vi "Begin.vi"(8 "error in":errorcluster) -> (0 "error out":errorcluster)   [LabVIEW 2014]
doc: "Called before other user functions, this VI is expected to open initial I/O refnums, load in file data, and do all program initialization. Notice that the <B>error out</B> terminal is simply used for data flow. Wiring it to other structures or subVIs ensures that this VI runs first."
uses:
  <vilib>/Rock Robotics/SystemInterfaces/DIO/FPGA_DIOPWMChannel.ctl
  <vilib>/Rock Robotics/WPI/SafetyOutput/WPI_SafetyOutputConfigMenu.ctl
  <vilib>/Rock Robotics/WPI/DriverStation/WPI_DriverStationRobotMode2.ctl
  <vilib>/Rock Robotics/WPI/Joystick/WPI_JoystickDeviceEnum.ctl
  <vilib>/Rock Robotics/SystemInterfaces/i2clib/i2c_bus.ctl
  <vilib>/Rock Robotics/SystemInterfaces/Typedef/FPGA_TypedefDigitalModule.ctl
  <vilib>/Rock Robotics/WPI/RobotDrive/WPI_RobotDriveOpen2MotorWithTalon.vi
  Robot Global Data.vi
  <vilib>/Rock Robotics/Network Tables/SD Write String Array.vi
panel:
  out "I2c Error":errorcluster
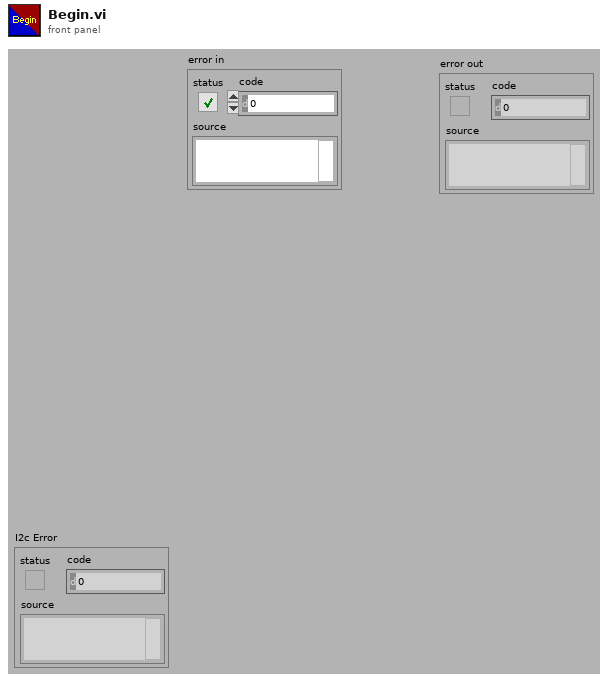
[diagram p1: front panel]
types:
  T1 = typedef "FPGA_TypedefDigitalModule.ctl" = enum16{"Controller 1"}
  T2 = typedef "i2c_bus.ctl" = enum16{"I2C On-Board", "I2C MXP", "Invalid"}
  T3 = typedef "WPI_JoystickDeviceEnum.ctl" = enum16{"USB 0", "USB 1", "USB 2", "USB 3", "USB 4", "USB 5"}
  T4 = typedef "WPI_DriverStationRobotMode2.ctl" = enum16{"Autonomous Disabled", "Autonomous Enabled", "Teleop Disabled", "Teleop Enabled", "Disconnected", "Finish", "Test Disabled", "Test Enabled", "Emergency Stopped"}
  T5 = typedef "WPI_SafetyOutputConfigMenu.ctl" = enum16{"Enable", "Disable"}
  T6 = typedef "FPGA_DIOPWMChannel.ctl" = enum8{"PWM 0", "PWM 1", "PWM 2", "PWM 3", "PWM 4", "PWM 5", "PWM 6", "PWM 7", "PWM 8", "PWM 9", "PWM MXP 0", "PWM MXP 1", "PWM MXP 2", "PWM MXP 3", "PWM MXP 4", "PWM MXP 5", "PWM MXP 6", "PWM MXP 7", "PWM MXP 8", "PWM MXP 9", "Invalid"}
  T7 = typedef "WPI_JoystickDevRef.ctl" = cluster{"Device":T3}
  T8 = typedef "WPI_RobotDriveDevRef.ctl" = cluster{"DevStatus":errorcluster, "Motors[]":T9[], "Square Inputs":bool, "Max Output":dbl}
  T9 = typedef "WPI_MotorControlDeviceRef.ctl" = cluster{"DeviceStatus":errorcluster, "Type":T10, "PWM":cluster{"Controller":T1, "PWM Channel":T6, "DeadBand":T11}, "CAN":cluster{"Device Number":u8, "Control Mode":T12, "Semaphore":T13, "Max Vout":dbl, "TalonSRX Control Mode":T14}, "Invert":bool, "TransformRef":T15, "InvTransformRef":T15}
  T10 = typedef "WPI_MotorControlType.ctl" = enum16{"PWM", "CAN", "CANTalonSRX"}
  T11 = typedef "WPI_PWMDeadband.ctl" = cluster{"Name":string, "maxPositivePwm":i32, "minPositivePwm":i32, "centerPwm":i32, "maxNegativePwm":i32, "minNegativePwm":i32, "angularRange":u16}
  T12 = typedef "WPI_CANJaguar_ControlMode.ctl" = enum8{"Percent VBus", "Current", "Speed", "Position", "Voltage"}
  T13 = typedef "Semaphore RefNum" = refnum<k1>
  T14 = typedef "WPI_CANTalonSRX_APIControlMode.ctl" = enum8{"Percent VBus", "Speed", "Position", "Slave", "Unchanged / Invalid"}
  T15 = typedef "WPI_PWMTransform_ConPane.ctl" = refnum<vi>
  T16 = typedef "WPI_I2CDevRef.ctl" = cluster{"DevStatus":errorcluster, "Controller":T1, "Device Address":u8, "Handle":i32, "I2C Bus":T2}
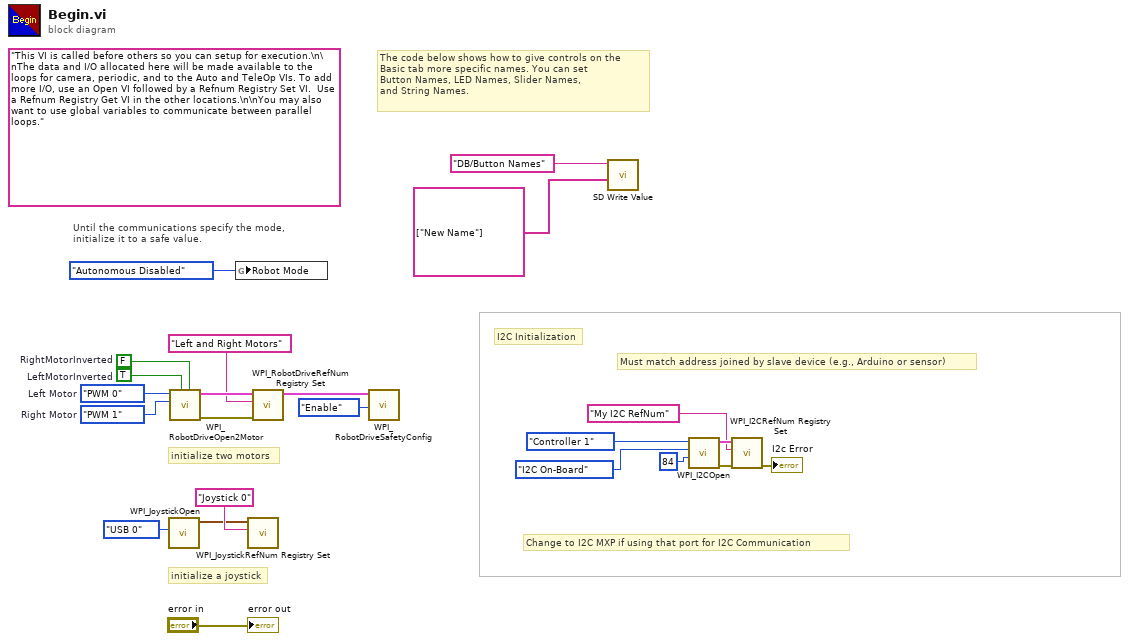
[diagram p0: block diagram]
diagram:
  (unwired) "This VI is called before others so you can setup for execution.\n\nThe data and I/O allocated here will be made available to the loops for camera, periodic, and to the Auto and TeleOp VIs. To add more I/O, use an Open VI followed by a Refnum Registry Set VI.  Use a Refnum Registry Get VI in the other locations.\n\nYou may also want to use global variables to communicate between parallel loops."
  w17 = FPGA_DIOPWMChannel."PWM 1"  # Right Motor
  w18 = FPGA_DIOPWMChannel."PWM 0"  # Left Motor
  w22 = TRUE  # LeftMotorInverted
  w23 = FALSE  # RightMotorInverted
  # "I2C Initialization"
  # "Must match address joined by slave device (e.g., Arduino or sensor)"
  # "Change to I2C MXP if using that port for I2C Communication"
  # "The code below shows how to give controls on the\nBasic tab more specific names. You can set\nButton Names, LED Names, Slider Names,\nand String Names."
  # "initialize a joystick"
  # "Until the communications specify the mode,\ninitialize it to a safe value."
  # "initialize two motors"
  n1 = call <vilib>:"WPI_JoystickOpen.vi"("JoystickDevice"=WPI_JoystickDeviceEnum."USB 0") -> ("JoystickDevRef"=w12:T7)  [unwired: 10 in]
  n2 = call-poly <vilib>:"WPI_RobotDriveOpen2Motor.vi"("Right Motor Inverted"=w23, "Left Motor Inverted"=w22, "Right Motor"=w17, "Left Motor"=w18) -> ("error out"=w19:errorcluster, "RobotDriveDevRef"=w21:T8)  [unwired: 1 in, 5 out]
  n3 = global write "Robot Global Data.vi" "Robot Mode"(WPI_DriverStationRobotMode2."Autonomous Disabled" ("Robot Mode")) -> ()
  n4 = call <vilib>:"WPI_JoystickRefNum Registry Set.vi"("refnum name"="Joystick 0", "JoystickDevRef"=w12) -> ()  [unwired: 8 in, 2 out]
  n5 = call <vilib>:"WPI_RobotDriveRefNum Registry Set.vi"("error in (no error)"=w19, "refnum name"="Left and Right Motors", "RobotDriveDevRef"=w21) -> ("RobotDriveDevRef"=w16:T8)  [unwired: 8 out]
  n6 = call <vilib>:"WPI_RobotDriveSafetyConfig.vi"("mode"=WPI_SafetyOutputConfigMenu."Enable", "RobotDriveDevRef"=w16) -> ()  [unwired: 8 in, 2 out]
  n7 = call-poly <vilib>:"SD Write Value.vi"("String Array"=string[] ["New Name"], "Name"="DB/Button Names") -> ()  [unwired: 8 in, 2 out]
  n8 = call <vilib>:"WPI_I2COpen.vi"("Device Address"=u8 84, "I2C Bus"=i2c_bus."I2C On-Board", "Controller"=FPGA_TypedefDigitalModule."Controller 1") -> ("error out"=w2:errorcluster, "I2CDevRef"=w4:T16)  [unwired: 7 in]
  n9 = call <vilib>:"WPI_I2CRefNum Registry Set.vi"("error in (no error)"=w2, "refnum name"="My I2C RefNum", "I2CDevRef"=w4) -> ("error out"=→"I2c Error":errorcluster)  [unwired: 7 in, 1 out]
  "error out" <- "error in"
